vi "Setting_OneRele.vi"(8 "data":bool, 11 "line":refnum<k21>) -> (0 "error out":errorcluster)   [LabVIEW 2023]
uses:
  <vilib>/ULx/Create Channel.llb/ULx Create Channel (DO-Digital Output).vi
  <vilib>/ULx/Write.llb/ULx Write (Digital Bool 1Line 1Point).vi
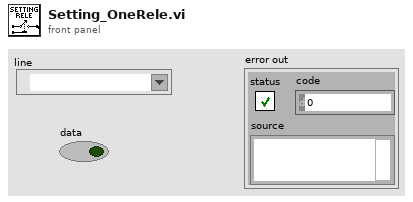
[diagram p1: front panel]
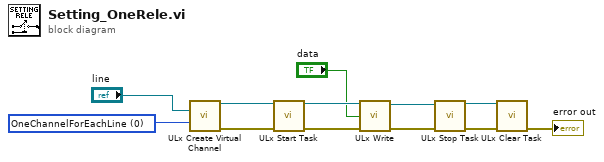
[diagram p0: block diagram]
diagram:
  w3 = 0 items=["OneChannelForEachLine", "OneChannelForAllLines"] ("line grouping")
  n1 = call-poly <vilib>:"ULx Create Virtual Channel.vi"("lines"="line", "line grouping"=w3) -> ("task out"=w11:refnum<k24>, "error out"=w12:errorcluster)  [unwired: 12 in]
  n2 = call <vilib>:"ULx Start Task.vi"("task in"=w11, "error in"=w12) -> ("task out"=w10:refnum<k24>, "error out"=w6:errorcluster)  [unwired: 12 in]
  n3 = call-poly <vilib>:"ULx Write.vi"("task in"=w10, "data"="data", "error in"=w6) -> ("task out"=w5:refnum<k24>, "error out"=w8:errorcluster)  [unwired: 10 in, 1 out]
  n4 = call <vilib>:"ULx Stop Task.vi"("error in"=w8, "task in"=w5) -> ("error out"=w9:errorcluster, "task out"=w4:refnum<k24>)  [unwired: 8 in]
  n5 = call <vilib>:"ULx Clear Task.vi"("task in"=w4, "error in"=w9) -> ("error out"=→"error out":errorcluster)  [unwired: 13 in]
